vi "Daq QPDs.vi"() -> ()   [LabVIEW 2018]
uses:
  <vilib>/Analysis/baseanly.llb/Mean (DBL).vi
  <vilib>/express/express analysis/Spectral/Block/exnSpectralBlock spectral measurements peak poly.vi
  <vilib>/express/express analysis/Spectral/Block/exnSpectralBlock spectral measurements peak DDT.vi
  <vilib>/express/express analysis/Spectral/XNode/ExpressSpectralMeasurementsBlockNode.xnode
  <vilib>/Analysis/NI_AALBase.lvlib
panel:
  in  "Filename 2":path=path "C:/Users/physics-svc-fulda/Desktop/LabVIEW Data/DC OFFset.lvm" caption="Filename"
  out "DC: A+B+C+D":dynamicdata(graph)
  out "Pout QPD":dbl
  out "X: (A+B)-(C+D)":dynamicdata(graph)
  out "DC - 4":dynamicdata(graph)
  out "RF - 4":dynamicdata(graph)
  out "RF: A+B+C+D":dynamicdata(graph)
  in  "X residual":dbl
  in  "Enable":bool=TRUE
  out "Saving Data 3":bool caption="Saving Data"
  in  "# of samples":i32=300
  in  "Y Upper Cut-Off":dbl=50.0 caption="Upper Cut-Off"
  out "Saving Data 2":bool caption="Saving Data"
  out "Filename Out 2":path caption="Filename Out"
  in  "Filename 4":path=path "C:/Users/physics-svc-fulda/Desktop/WFS_RF.lvm" caption="Filename"
  in  "Enable 2":bool=TRUE caption="Enable"
  out "X Signal Peak Value":dbl
  out "X Peak/Pout":dbl
  out "Pout":dbl
  in  "PD Offset":dbl
  out "Pout":dynamicdata(graph)
  in  "Filename 3":path=path "C:/Users/physics-svc-fulda/Desktop/LabVIEW Data/RF OFFset.lvm"
  out "RF Offset A":dbl format="%0.6f"
  out "RF Offset C":dbl format="%0.6f"
  out "RF Offset B":dbl format="%0.6f"
  out "RF Offset D":dbl format="%0.6f"
  out "A":dynamicdata(graph)
  out "DC Offset A":dbl format="%0.6f"
  out "DC Offset C":dbl format="%0.6f"
  out "DC Offset B":dbl format="%0.6f"
  out "DC Offset D":dbl format="%0.6f"
  out "RF Responsivity D":dbl
  out "RF Responsivity C":dbl
  out "RF Responsivity B":dbl
  out "RF Responsivity A":dbl
  out "DC Responsivity D":dbl
  out "DC Responsivity C":dbl
  out "DC Responsivity B":dbl
  out "DC Responsivity A":dbl
  out "X/Y":dbl
  out "Y Signal Peak Value":dbl
  in  "X Upper Cut-Off":dbl=50.0 caption="Upper Cut-Off"
  in  "X Lower Cut-Off":dbl=1.0 caption="Lower Cut-Off"
  out "X FFT":dynamicdata(graph)
  in  "Y Lower Cut-Off":dbl=1.0 caption="Lower Cut-Off"
  out "Y FFT":dynamicdata(graph)
  out "Y: (A+C)-(B+D)":dynamicdata(graph)
  out "RF: L-R":dynamicdata(graph)
  out "D":dynamicdata(graph)
  out "B":dynamicdata(graph)
  out "C":dynamicdata(graph)
  in  "STOP":bool
  out "Beam Centering":cluster{"Y":dbl[], "Y":dbl[]}[](graph)
  out "Y: (A+C)-(B+D)":dynamicdata(graph)
  out "X: (A+B)-(C+D)":dynamicdata(graph)
  out "Filename Out":path
  in  "Filename":path=path "C:/Users/physics-svc-fulda/Desktop/Data.lvm"
  out "D":dynamicdata(graph)
  out "B":dynamicdata(graph)
  out "C":dynamicdata(graph)
  out "A":dynamicdata(graph)
  in  "timeout (s)":dbl=10.0 format="%0.2f"
  in  "rate":dbl=1000.0
  # "DC"
  # "RF"
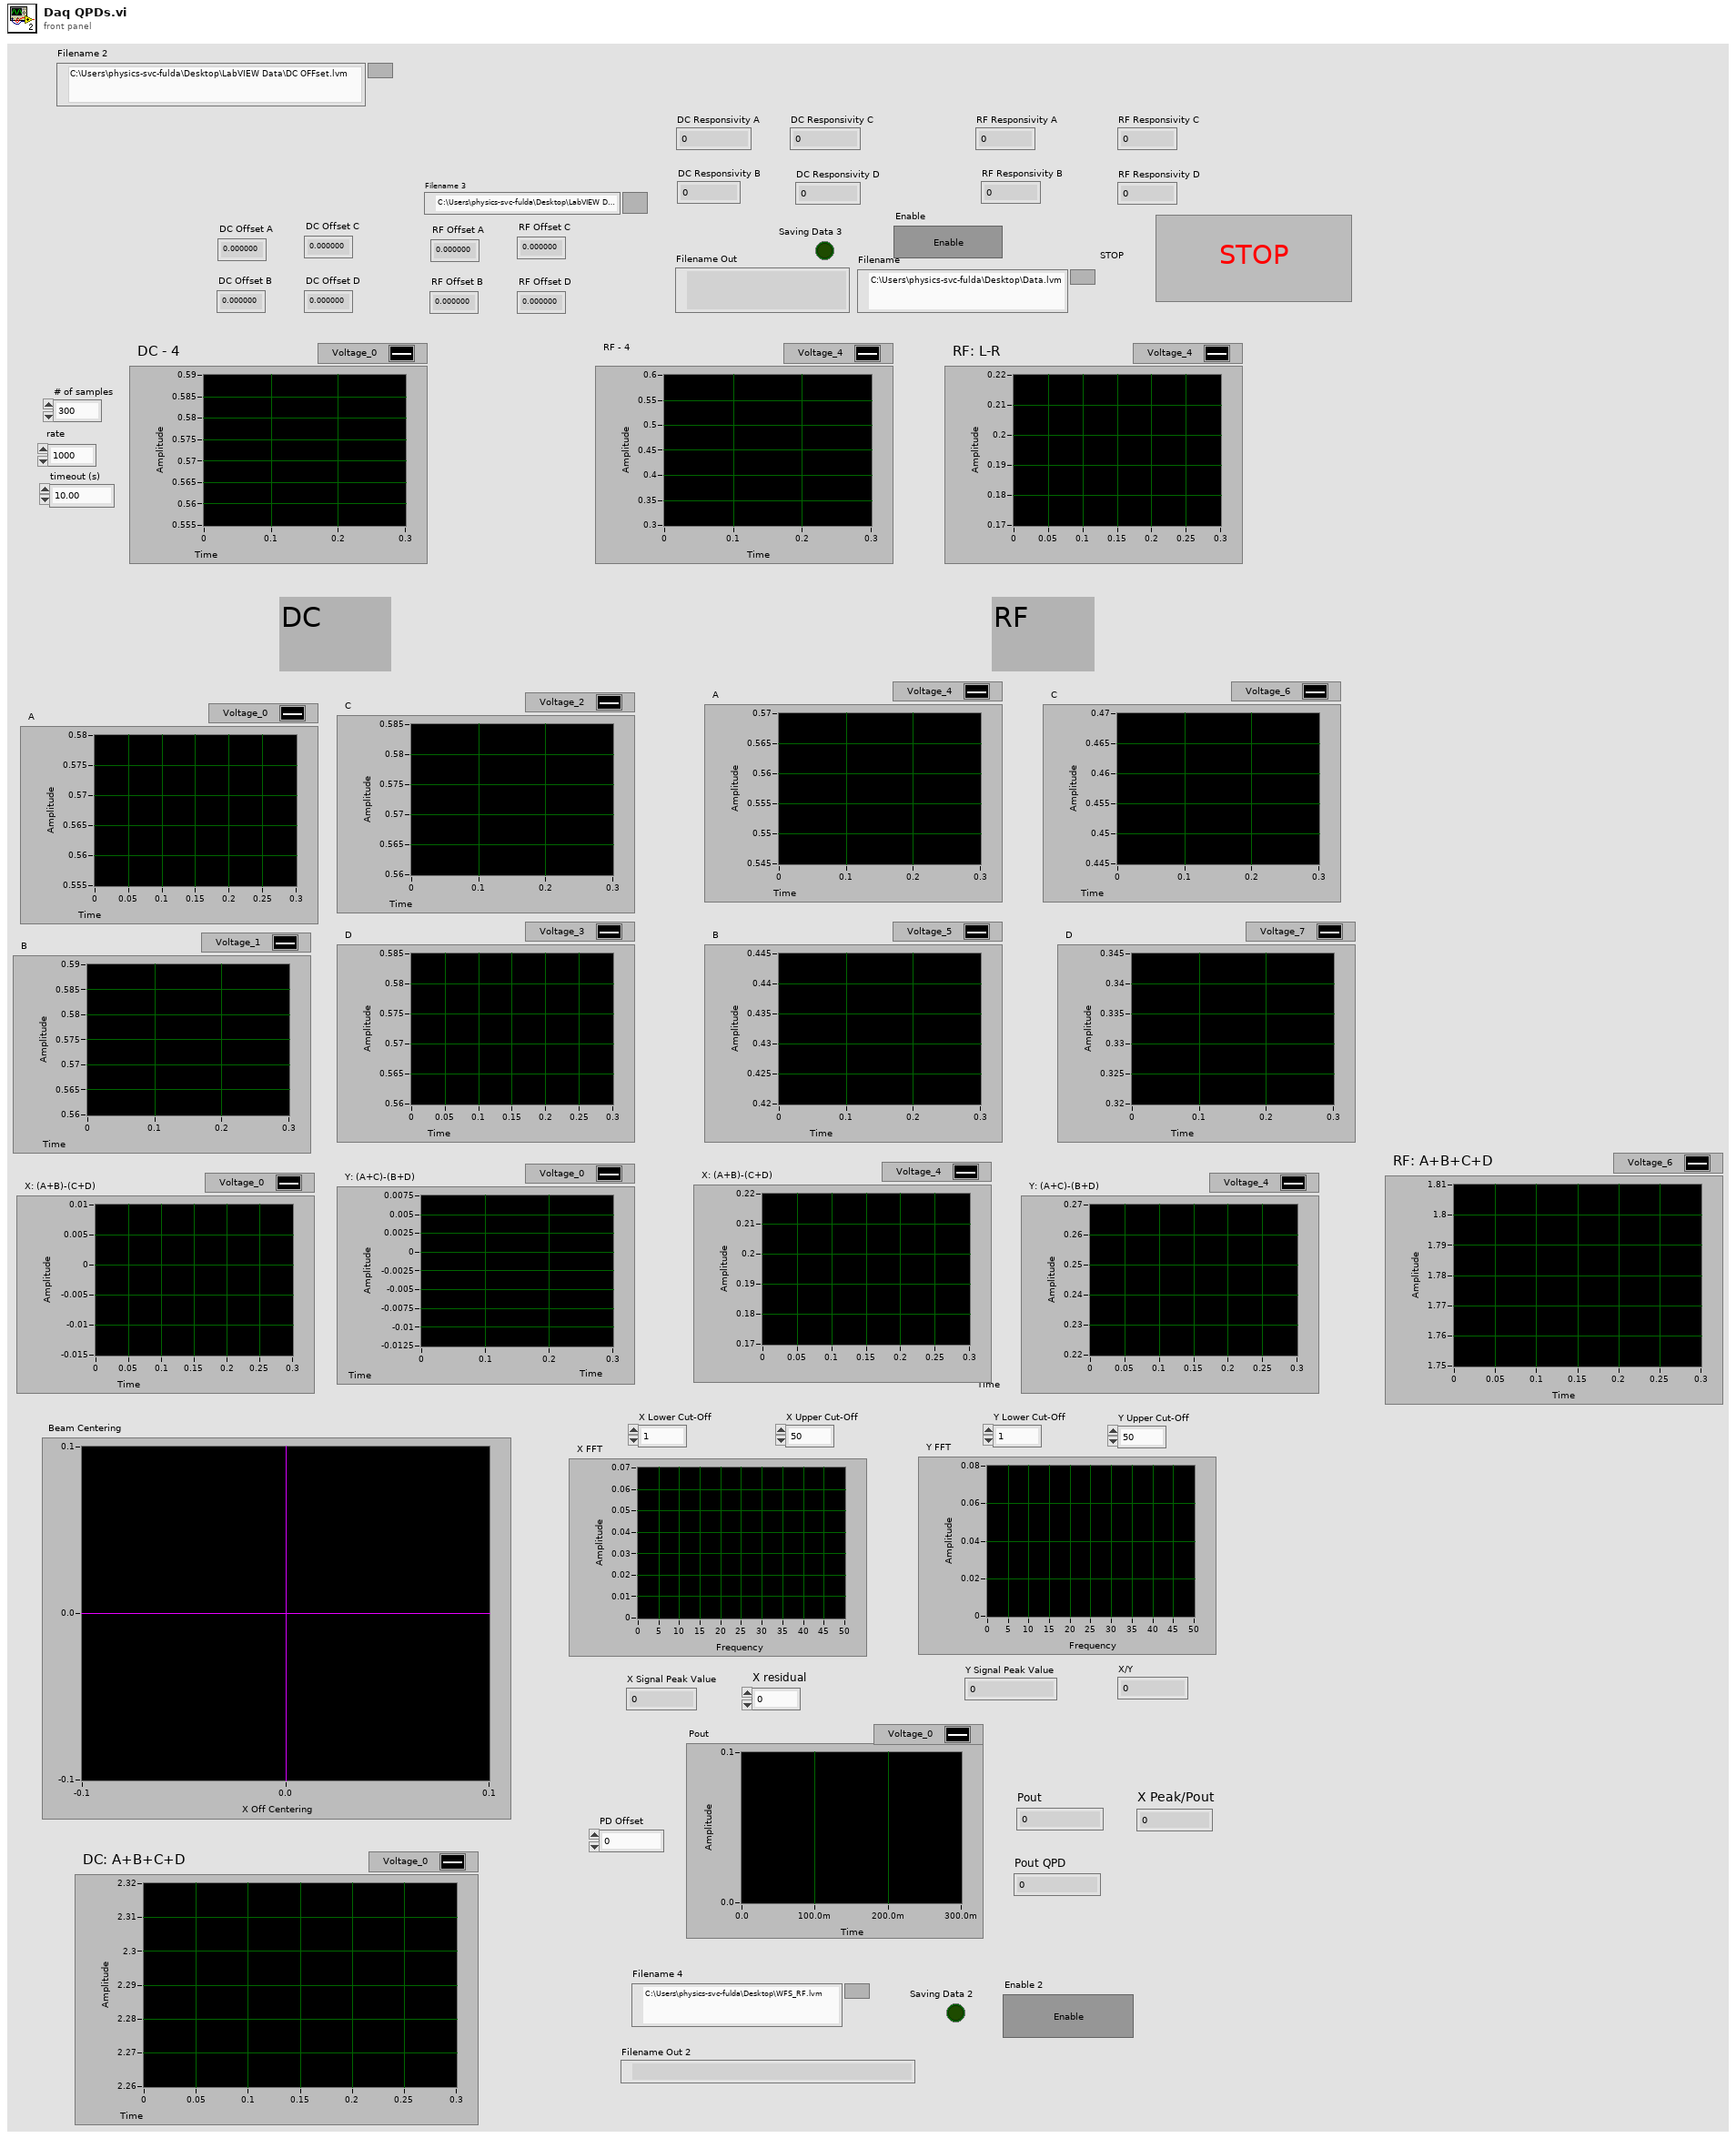
[diagram p1: front panel]
types:
  T1 = cluster{"averaging mode":u16, "weighting mode":u16, "number of averages":u32}
  T2 = cluster{"dB On (F)":bool, "unwrap phase (F)":bool, "convert to degree (F)":bool}
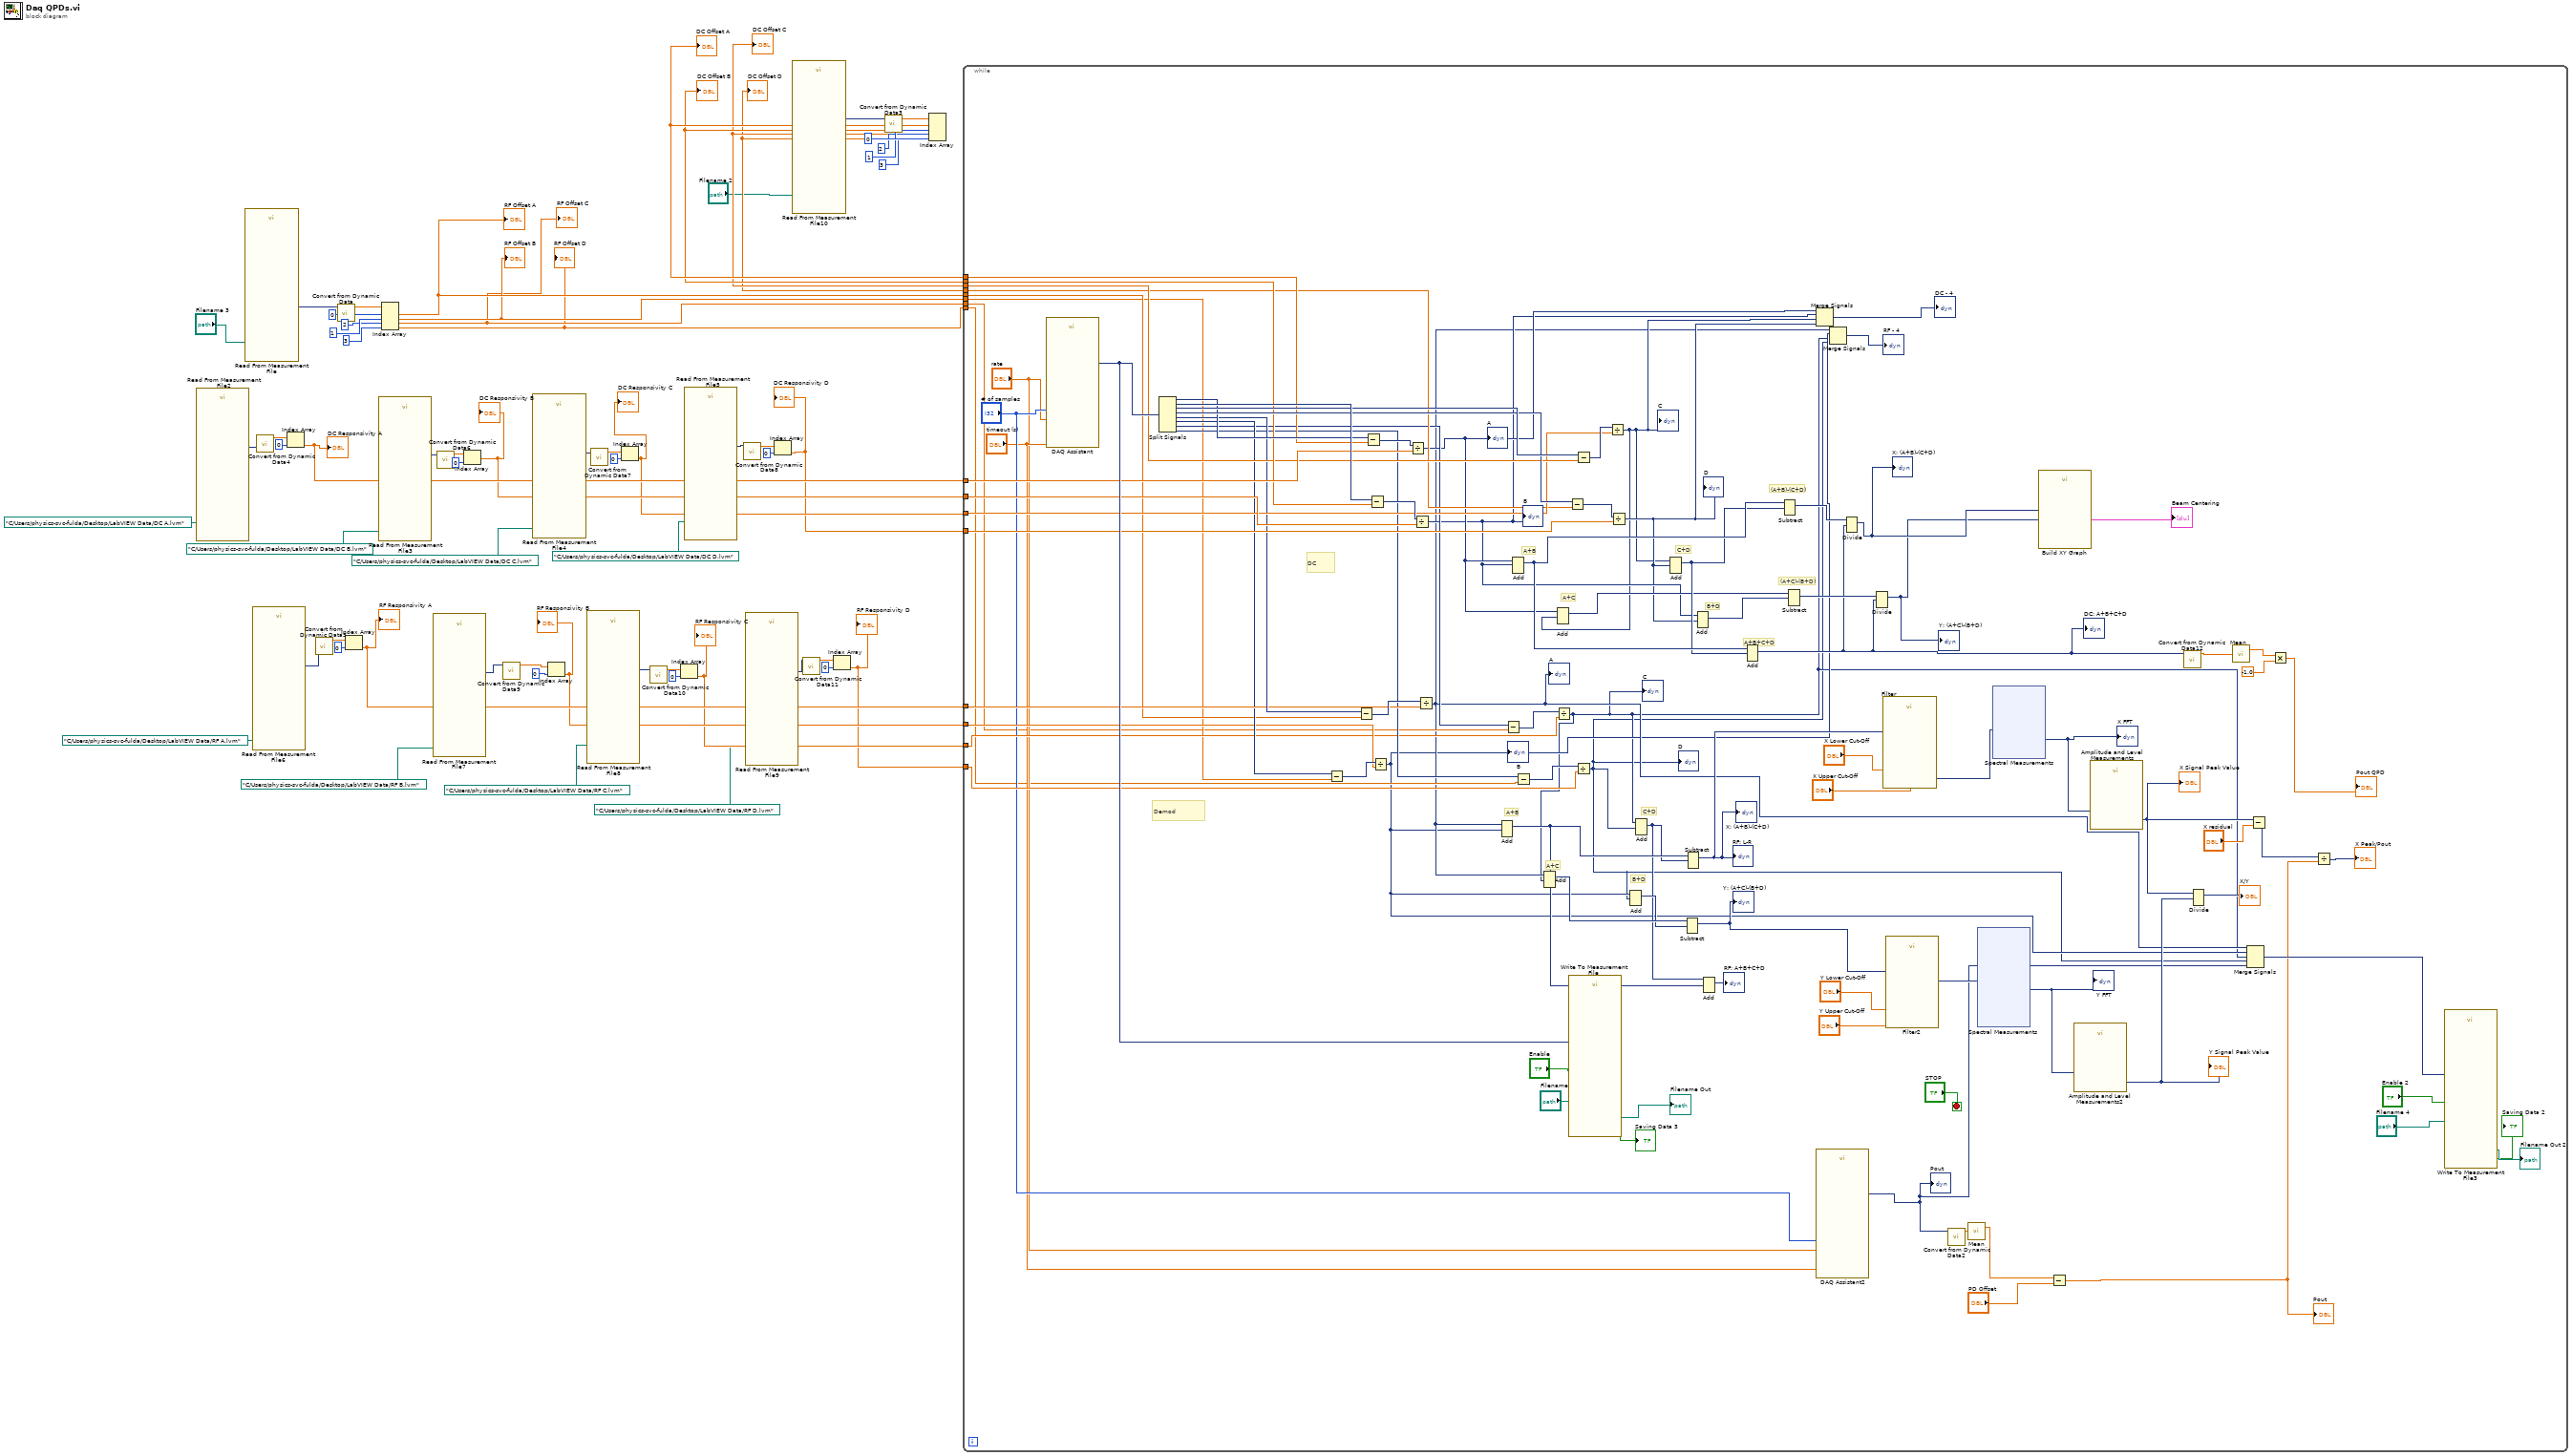
[diagram p0: block diagram]
diagram:
  n1 = call "Read From Measurement File2"("Filename"=path "C:/Users/physics-svc-fulda/Desktop/LabVIEW Data/DC A.lvm") -> ("Signals"=w47:dynamicdata)  [unwired: 5 in, 5 out]
  n2 = call "Read From Measurement File"("Filename"="Filename 3") -> ("Signals"=w11:dynamicdata)  [unwired: 5 in, 5 out]
  n3 = call "Read From Measurement File6"("Filename"=path "C:/Users/physics-svc-fulda/Desktop/LabVIEW Data/RF A.lvm") -> ("Signals"=w50:dynamicdata)  [unwired: 5 in, 5 out]
  n4 = call "Convert from Dynamic Data4"("Dynamic Data Type"=w47) -> ("Array"=w48:dbl[])  [unwired: 3 in]
  n5 = Index Array(array=w48, index=0) -> (element=w32:dbl)
  "DC Responsivity A" <- w32
  n6 = call "Convert from Dynamic Data5"("Dynamic Data Type"=w50) -> ("Array"=w49:dbl[])  [unwired: 3 in]
  n7 = call "Convert from Dynamic Data"("Dynamic Data Type"=w11) -> ("Array"=w12:dbl[])  [unwired: 3 in]
  n8 = Index Array(array=w49, index=0) -> (element=w28:dbl)
  "RF Responsivity A" <- w28
  n9 = call "Read From Measurement File3"("Filename"=path "C:/Users/physics-svc-fulda/Desktop/LabVIEW Data/DC B.lvm") -> ("Signals"=w52:dynamicdata)  [unwired: 5 in, 5 out]
  n10 = Index Array(array=w12, index #1=0 ("index"), index #2=1 ("index"), index #3=2 ("index"), index #4=3 ("index")) -> (element #1=w6:dbl, element #2=w5:dbl, element #3=w4:dbl, element #4=w3:dbl)
  "RF Offset D" <- w3
  "RF Offset B" <- w5
  "RF Offset C" <- w4
  "RF Offset A" <- w6
  n11 = call "Read From Measurement File7"("Filename"=path "C:/Users/physics-svc-fulda/Desktop/LabVIEW Data/RF B.lvm") -> ("Signals"=w39:dynamicdata)  [unwired: 5 in, 5 out]
  n12 = call "Convert from Dynamic Data6"("Dynamic Data Type"=w52) -> ("Array"=w51:dbl[])  [unwired: 3 in]
  n13 = Index Array(array=w51, index=0) -> (element=w31:dbl)
  "DC Responsivity B" <- w31
  n14 = call "Convert from Dynamic Data9"("Dynamic Data Type"=w39) -> ("Array"=w41:dbl[])  [unwired: 3 in]
  n15 = call "Read From Measurement File4"("Filename"=path "C:/Users/physics-svc-fulda/Desktop/LabVIEW Data/DC C.lvm") -> ("Signals"=w54:dynamicdata)  [unwired: 5 in, 5 out]
  n16 = Index Array(array=w41, index=0) -> (element=w27:dbl)
  "RF Responsivity B" <- w27
  n17 = call "Read From Measurement File8"("Filename"=path "C:/Users/physics-svc-fulda/Desktop/LabVIEW Data/RF C.lvm") -> ("Signals"=w34:dynamicdata)  [unwired: 5 in, 5 out]
  n18 = call "Convert from Dynamic Data7"("Dynamic Data Type"=w54) -> ("Array"=w53:dbl[])  [unwired: 3 in]
  n19 = Index Array(array=w53, index=0) -> (element=w30:dbl)
  "DC Responsivity C" <- w30
  n20 = call "Convert from Dynamic Data10"("Dynamic Data Type"=w34) -> ("Array"=w38:dbl[])  [unwired: 3 in]
  n21 = Index Array(array=w38, index=0) -> (element=w26:dbl)
  "RF Responsivity C" <- w26
  n22 = call "Read From Measurement File5"("Filename"=path "C:/Users/physics-svc-fulda/Desktop/LabVIEW Data/DC D.lvm") -> ("Signals"=w56:dynamicdata)  [unwired: 5 in, 5 out]
  n23 = call "Convert from Dynamic Data8"("Dynamic Data Type"=w56) -> ("Array"=w55:dbl[])  [unwired: 3 in]
  n24 = call "Read From Measurement File9"("Filename"=path "C:/Users/physics-svc-fulda/Desktop/LabVIEW Data/RF D.lvm") -> ("Signals"=w33:dynamicdata)  [unwired: 5 in, 5 out]
  n25 = Index Array(array=w55, index=0) -> (element=w29:dbl)
  "DC Responsivity D" <- w29
  n26 = call "Read From Measurement File10"("Filename"="Filename 2") -> ("Signals"=w61:dynamicdata)  [unwired: 5 in, 5 out]
  n27 = call "Convert from Dynamic Data11"("Dynamic Data Type"=w33) -> ("Array"=w36:dbl[])  [unwired: 3 in]
  n28 = Index Array(array=w36, index=0) -> (element=w25:dbl)
  "RF Responsivity D" <- w25
  n29 = call "Convert from Dynamic Data3"("Dynamic Data Type"=w61) -> ("Array"=w62:dbl[])  [unwired: 3 in]
  n30 = Index Array(array=w62, index #1=0 ("index"), index #2=1 ("index"), index #3=2 ("index"), index #4=3 ("index")) -> (element #1=w24:dbl, element #2=w23:dbl, element #3=w22:dbl, element #4=w21:dbl)
  "DC Offset D" <- w21
  "DC Offset B" <- w23
  "DC Offset C" <- w22
  "DC Offset A" <- w24
  n31 = while {
    tunnel: w24 -> [w135]
    tunnel: w23 -> [w133]
    tunnel: w22 -> [w131]
    tunnel: w21 -> [w129]
    tunnel: w6 -> [w95]
    tunnel: w5 -> [w94]
    tunnel: w4 -> [w93]
    tunnel: w3 -> [w92]
    tunnel: w32 -> [w134]
    tunnel: w31 -> [w132]
    tunnel: w30 -> [w130]
    tunnel: w29 -> [w128]
    tunnel: w28 -> [w125]
    tunnel: w27 -> [w118]
    tunnel: w26 -> [w117]
    tunnel: w25 -> [w116]
    stop <- "STOP" stop-if-true
    # "B+D"
    # "A+C"
    # "C+D"
    # "A+B"
    # "(A+C)-(B+D)"
    # "(A+B)-(C+D)"
    # "A+B+C+D"
    # "B+D"
    # "A+C"
    # "C+D"
    # "A+B"
    # "Demod"
    # "DC"
    n32 = call "DAQ Assistant"("rate"="rate", "number of samples"="# of samples", "timeout (s)"="timeout (s)") -> ("data"=w155:dynamicdata)  [unwired: 14 in, 2 out]
    n33 = Split Signals(w155) -> (w137:dynamicdata, w147:dynamicdata, w145:dynamicdata, w143:dynamicdata, w127:dynamicdata, w123:dynamicdata, w121:dynamicdata, w119:dynamicdata)  [unwired: 8 in]
    n34 = Subtract(x=w123, y=w94) -> (x-y=w124:dynamicdata)
    n35 = Subtract(x=w127, y=w95) -> (x-y=w126:dynamicdata)
    n36 = Subtract(x=w137, y=w135) -> (x-y=w136:dynamicdata)
    n37 = Subtract(x=w147, y=w133) -> (x-y=w146:dynamicdata)
    n38 = Divide(x=w124, y=w118) -> (x/y=w65:dynamicdata)
    "B" <- w65
    n39 = Divide(x=w136, y=w134) -> (x/y=w80:dynamicdata)
    "A" <- w80
    n40 = Divide(x=w146, y=w132) -> (x/y=w79:dynamicdata)
    "B" <- w79
    n41 = Divide(x=w126, y=w125) -> (x/y=w66:dynamicdata)
    "A" <- w66
    n42 = Add(1:w65, 2:w66) -> (0:w83:dynamicdata)  [unwired: 1 in, 1 out]
    n43 = Subtract(x=w121, y=w93) -> (x-y=w122:dynamicdata)
    n44 = Add(1:w79, 2:w80) -> (0:w141:dynamicdata)  [unwired: 1 in, 1 out]
    n45 = Subtract(x=w119, y=w92) -> (x-y=w120:dynamicdata)
    n46 = Divide(x=w122, y=w117) -> (x/y=w64:dynamicdata)
    "C" <- w64
    n47 = Add(1:w64, 2:w66) -> (0:w115:dynamicdata)  [unwired: 1 in, 1 out]
    n48 = Subtract(x=w143, y=w129) -> (x-y=w142:dynamicdata)
    n49 = call "Write To Measurement File"("Signals"=w155, "Enable"="Enable", "Filename"="Filename") -> ("Filename Out"=→"Filename Out":path, "Saving Data"=→"Saving Data 3":bool)  [unwired: 14 in, 1 out]
    n50 = Divide(x=w120, y=w116) -> (x/y=w63:dynamicdata)
    "D" <- w63
    n51 = Subtract(x=w145, y=w131) -> (x-y=w144:dynamicdata)
    n52 = Divide(x=w144, y=w130) -> (x/y=w77:dynamicdata)
    "C" <- w77
    n53 = Add(1:w77, 2:w80) -> (0:w139:dynamicdata)  [unwired: 1 in, 1 out]
    n54 = Divide(x=w142, y=w128) -> (x/y=w78:dynamicdata)
    "D" <- w78
    n55 = Add(1:w63, 2:w65) -> (0:w114:dynamicdata)  [unwired: 1 in, 1 out]
    n56 = Add(1:w63, 2:w64) -> (0:w82:dynamicdata)  [unwired: 1 in, 1 out]
    n57 = Add(1:w78, 2:w77) -> (0:w140:dynamicdata)  [unwired: 1 in, 1 out]
    n58 = Subtract(1:w114, 2:w115) -> (0:w113:dynamicdata)  [unwired: 1 in, 1 out]
    "Y: (A+C)-(B+D)" <- w113
    n59 = Subtract(1:w82, 2:w83) -> (0:w73:dynamicdata)  [unwired: 1 in, 1 out]
    "RF: L-R" <- w73
    "X: (A+B)-(C+D)" <- w73
    n60 = Add(1:w78, 2:w79) -> (0:w138:dynamicdata)  [unwired: 1 in, 1 out]
    n61 = Add(1:w83, 2:w82) -> (0:→"RF: A+B+C+D":dynamicdata)  [unwired: 1 in, 1 out]
    n62 = Add(1:w140, 2:w141) -> (0:w71:dynamicdata)  [unwired: 1 in, 1 out]
    "DC: A+B+C+D" <- w71
    n63 = Subtract(1:w140, 2:w141) -> (0:w110:dynamicdata)  [unwired: 1 in, 1 out]
    n64 = Subtract(1:w138, 2:w139) -> (0:w109:dynamicdata)  [unwired: 1 in, 1 out]
    n65 = Merge Signals(w80, w79, w77, w78) -> (→"DC - 4":dynamicdata)
    n66 = call "DAQ Assistant2"("rate"="rate", "number of samples"="# of samples", "timeout (s)"="timeout (s)") -> ("data"=w74:dynamicdata)  [unwired: 14 in, 2 out]
    "Pout" <- w74
    n67 = Merge Signals(w66, w65, w64, w63) -> (→"RF - 4":dynamicdata)
    n68 = Divide(1:w71, 2:w110) -> (0:w85:dynamicdata)  [unwired: 1 in, 1 out]
    "X: (A+B)-(C+D)" <- w85
    n69 = Divide(1:w71, 2:w109) -> (0:w84:dynamicdata)  [unwired: 1 in, 1 out]
    "Y: (A+C)-(B+D)" <- w84
    n70 = call "Filter"("Lower Cut-Off"="X Lower Cut-Off", "Upper Cut-Off"="X Upper Cut-Off", "Signal"=w73) -> ("Filtered Signal"=w152:dynamicdata)  [unwired: 7 in, 1 out]
    n71 = call "Filter2"("Lower Cut-Off"="Y Lower Cut-Off", "Upper Cut-Off"="Y Upper Cut-Off", "Signal"=w113) -> ("Filtered Signal"=w154:dynamicdata)  [unwired: 7 in, 1 out]
    n72 = call "Convert from Dynamic Data2"("Dynamic Data Type"=w74) -> ("Array"=w104:dbl[])  [unwired: 3 in]
    n73 = call-poly <vilib>:"Mean.vi"("X"=w104) -> ("mean"=w103:dbl)  [unwired: 1 out]
    n74 = xnode "Spectral Measurements"("Signals"=w154) -> ("FFT - (Peak)"=w111:dynamicdata)  [unwired: 1 in, 2 out]
    "Y FFT" <- w111
    n75 = xnode "Spectral Measurements"("Signals"=w152) -> ("FFT - (Peak)"=w112:dynamicdata)  [unwired: 1 in, 2 out]
    "X FFT" <- w112
    n76 = call "Build XY Graph"("Y Input"=w84, "X Input"=w85) -> ("XY Graph"=→"Beam Centering":cluster{"X":dbl[], "Y":dbl[]}[])  [unwired: 8 in, 1 out]
    n77 = Subtract(x=w103, y="PD Offset") -> (x-y=w67:dbl)
    "Pout" <- w67
    n78 = call "Amplitude and Level Measurements2"("Signals"=w111) -> ("Positive Peak"=w108:dynamicdata)  [unwired: 13 in, 1 out]
    "Y Signal Peak Value" <- w108
    n79 = call "Amplitude and Level Measurements"("Signals"=w112) -> ("Positive Peak"=w87:dynamicdata)  [unwired: 13 in, 1 out]
    "X Signal Peak Value" <- w87
    n80 = call "Convert from Dynamic Data12"("Dynamic Data Type"=w71) -> ("Array"=w72:dbl[])  [unwired: 3 in]
    n81 = Divide(1:w108, 2:w87) -> (0:→"X/Y":dynamicdata)  [unwired: 1 in, 1 out]
    n82 = call-poly <vilib>:"Mean.vi"("X"=w72) -> ("mean"=w70:dbl)  [unwired: 1 out]
    n83 = Merge Signals(w66, w65, w64, w63, w74) -> (w100:dynamicdata)
    n84 = Subtract(x=w87, y="X residual") -> (x-y=w86:dynamicdata)
    n85 = Multiply(x=w70, y=-1.0) -> (x*y=→"Pout QPD":dbl)
    n86 = Divide(x=w86, y=w67) -> (x/y=→"X Peak/Pout":dynamicdata)
    n87 = call "Write To Measurement File3"("Signals"=w100, "Enable"="Enable 2", "Filename"="Filename 4") -> ("Filename Out"=→"Filename Out 2":path, "Saving Data"=→"Saving Data 2":bool)  [unwired: 14 in, 1 out]
  }
